vi "savComDataFits_FGV.vi"(8 "InError":errorcluster caption="entrée d'erreur (pas d'erreur)", 9 "Cluster":T1={"file (use dialog)"=path "", "Type de données"=enum."SGL (float 32bit)", "Commentaire"="", "naxis1"=0, "naxis2"=0, "naxis3"=0, "Exptime"=1.0}, 10 "SGL 32 bits":sgl[](array[numeric]), 11 "Énum":T3) -> (0 "sortie d'erreur":errorcluster)   [LabVIEW 2020]
uses:
  BigDataFits.ctl
  ClustBigFilFits.ctl
  DataTyp_Header.ctl
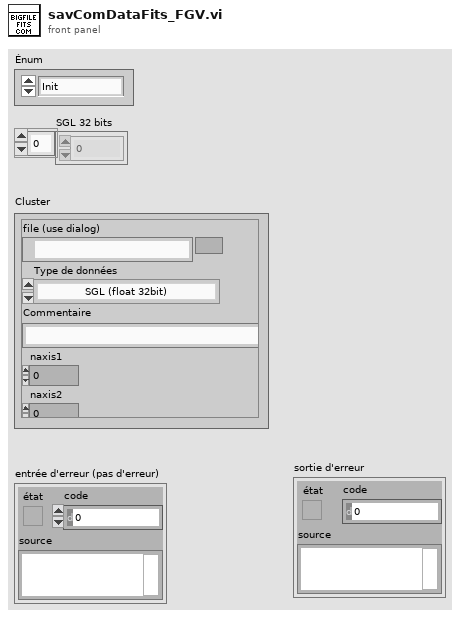
[diagram p1: front panel]
types:
  T1 = typedef "ClustBigFilFits.ctl" = cluster{"file (use dialog)":path, "Type de données":T2, "Commentaire":string, "naxis1":i32, "naxis2":i32, "naxis3":i32, "Exptime":sgl}
  T2 = typedef "DataTyp_Header.ctl" = enum16{"U8 (unsigned integer 8bit)", "I16 (signed integer 16bit)", "U16 (unsigned integer 16 bit)", "I32 (signed integer 32bit)", "U32 (unsigned integer 32 bit)", "SGL (float 32bit)", "DBL(float 64bit)", "complex (2xfloat 64bit)"}
  T3 = typedef "BigDataFits.ctl" = enum16{"Init", "WritHeader", "WritData", "Close"}
  T4 = enum16{"open", "replace", "create", "open or create", "replace or create", "replace or create with confirmation"}
  T5 = enum16{"big-endian, network order", "native, host order", "little-endian"}
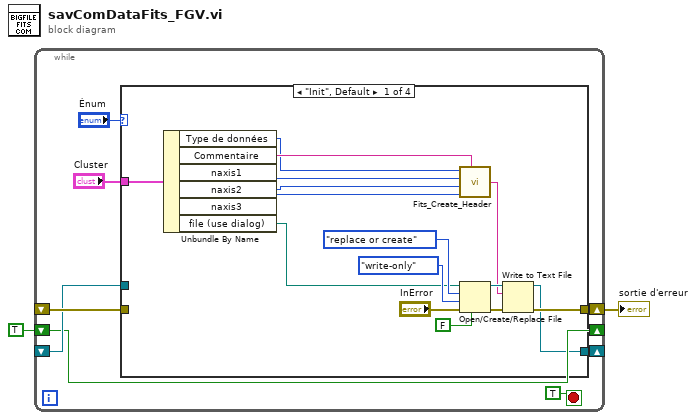
[diagram p0: block diagram]
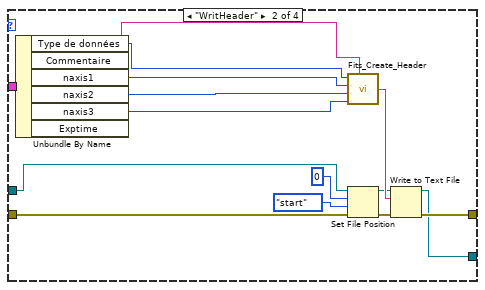
[diagram p2: hidden frame]
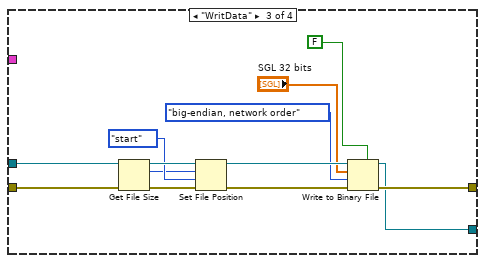
[diagram p3: hidden frame]
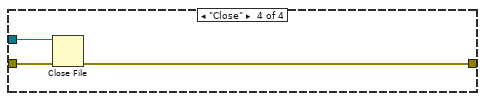
[diagram p4: hidden frame]
diagram:
  n1 = while {
    shift-right: [w3] -> _
    shift-left: TRUE -> [w3]
    shift-right: [w7] -> _
    shift-left: _ -> [w5]
    shift-right: [w8] -> w2
    shift-left: _ -> [w6]
    stop <- TRUE stop-if-true
    n2 = case shown="\"Init\", Default" "Énum" {
      tunnel: [w20 w40 w44 w56] -> w8
      tunnel: [w19 w39 w43 _] -> w7
      tunnel: w6 -> [_ w35 w46 w57]
      tunnel: w5 -> [_ w34 w45 w55]
      tunnel: "Cluster" -> [w18 w32 _ _]
      frame "Init", Default {
        n3 = Unbundle By Name(w18) -> ("Type de données"=w12:T2, "Commentaire"=w16:string, "naxis1"=w15:i32, "naxis2"=w14:i32, "naxis3"=w13:i32, "file (use dialog)"=w17:path)
        n4 = call "Fits_Create_Header.vi"("Commentaire"=w16, "naxis3"=w13, "naxis2"=w14, "naxis1"=w15, "Type de données"=w12) -> ("FITS header"=w21:string)  [unwired: 1 in]
        n5 = Open/Create/Replace File(file path (use dialog)=w17, error in="InError", operation (0:open)=T4."replace or create" ("opération (0 : open)"), access (0:read/write)=enum16{"read/write", "read-only", "write-only"}."write-only" ("accès (0 : read/write)"), disable buffering (F)=FALSE) -> (refnum out=w22:refnum<file>, error out=w23:errorcluster)  [unwired: 1 in, 1 out]
        n6 = Write to Text File(file (use dialog)=w22, text=w21, error in=w23) -> (refnum out=w19:refnum<file>, error out=w20:errorcluster)  [unwired: 1 in, 1 out]
      }
      frame "WritHeader" {
        n7 = Unbundle By Name(w32) -> ("Type de données"=w27:T2, "Commentaire"=w31:string, "naxis1"=w28:i32, "naxis2"=w29:i32, "naxis3"=w30:i32)  [unwired: 1 out]
        n8 = call "Fits_Create_Header.vi"("Commentaire"=w31, "naxis3"=w30, "naxis2"=w29, "naxis1"=w28, "Type de données"=w27) -> ("FITS header"=w41:string)  [unwired: 1 in]
        n9 = Set File Position(offset (in bytes) (0)=i64 0 ("offset (en octets) (0)"), refnum=w34, from (0:start)=enum16{"start", "end", "current"}."start" ("à partir de (0 : start)"), error in=w35) -> (refnum out=w33:refnum<file>, error out=w36:errorcluster)
        n10 = Write to Text File(file (use dialog)=w33, text=w41, error in=w36) -> (refnum out=w39:refnum<file>, error out=w40:errorcluster)  [unwired: 1 in, 1 out]
      }
      frame "WritData" {
        n11 = Get File Size(file=w45, error in=w46) -> (refnum out=w54:refnum<file>, size (in bytes)=w51:i64, 0:w52:errorcluster)
        n12 = Set File Position(offset (in bytes) (0)=w51, refnum=w54, from (0:start)=enum16{"start", "end", "current"}."start" ("à partir de (0 : start)"), error in=w52) -> (refnum out=w49:refnum<file>, error out=w50:errorcluster)
        n13 = Write to Binary File(file (use dialog)=w49, data="SGL 32 bits", error in=w50, 5:FALSE ("ajouter une taille de tableau ou de chaîne ? (V)"), 9:T5."big-endian, network order" ("ordre des octets (0 : big-Endian, network order)")) -> (refnum out=w43:refnum<file>, error out=w44:errorcluster)  [unwired: 1 in, 1 out]
      }
      frame "Close" {
        n14 = Close File(refnum=w55, error in=w57) -> (error out=w56:errorcluster)  [unwired: 1 out]
      }
    }
  }
  "sortie d'erreur" <- w2
